vi "sample4(Multi).vi"() -> ()   [LabVIEW 2011]
uses:
  <vilib>/Platform/TimedLoop/XDataNode/timing_clust.ctl
  <vilib>/Platform/TimedLoop/XDataNode/nitl_modes.ctl
  <vilib>/Platform/TimedLoop/XDataNode/wakeup.ctl
  <vilib>/Platform/TimedLoop/XDataNode/XDataNode.xnode
  <vilib>/Platform/TimedLoop/XDataNode/XDNodeRunTimeDep.lvlib
panel:
  out "err":errorcluster caption="エラー出力" {"code" format="%04x"}
  in  "OffsetTime":u32=20
  in  "frequency":dbl=0.3
  in  "waveform":enum16{"sin", "square"}(ring)
  in  "Target ID":u8=1 max=253
  in  "Baudrate":u32=1000000
  in  "COM":refnum<visa-resource-name> caption="COMポート"
  in  "10/12bit":bool
  out "present load":i32
  in  "wave":bool
  out "CtrlTable":u8[](array[numeric]) format="%02x"
  out "Chart":T1(graph)
  out "STOP2":bool
  out "present position":u16
  in  "STOP":bool
  in  "goal position":u16(knob) scale=0.0..1023.0
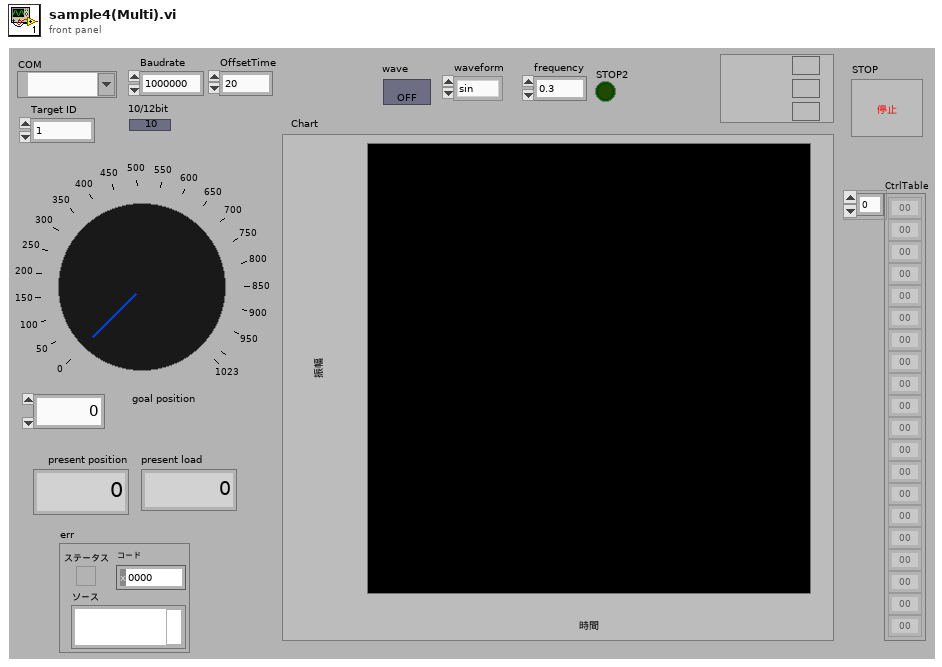
[diagram p1: front panel]
types:
  T1 = cluster{"pos":u16, "present pos":u16, "load":i32}
  T2 = typedef "XDNodeRunTimeDep.lvlib/timing_clust.ctl" = cluster{"Expected End [f-1]":u64, "Actual End [f-1]":u64, "Finished Late? [f-1]":bool, "Expected End [i-1]":u64, "Actual End [i-1]":u64, "Finished Late? [i-1]":bool, "Expected Start [i]":u64, "Actual Start [i]":u64, "Expected Start [f]":u64, "Actual Start [f]":u64, "Source Name":string, "Structure Name":string, "Period":i64, "Deadline":i64, "Offset":i64, "Start":i64, "Priority":i32, "Timeout":i32, "Mode":T3, "Wakeup Reason":T4, "Error":errorcluster, "Source Type":string, "Secondary Source Type":string, "Global End Time":u64, "Global Start Time":u64, "Frame Duration":u64, "Iteration Duration":u64, "Assigned CPU":i32, "I/O Scan Engine Mode":u32}
  T3 = typedef "XDNodeRunTimeDep.lvlib/nitl_modes.ctl" = enum32{"No Change", "Process missed periods, maintain original phase", "Discard missed periods, maintain original phase", "Process missed periods, ignore original phase", "Discard missed periods, ignore original phase"}
  T4 = typedef "XDNodeRunTimeDep.lvlib/wakeup.ctl" = enum32{"Normal", "Aborted", "Asynchronous wakeup", "Timing source error", "Timed loop error", "Timeout"}
  T5 = cluster{"goal position":u16, "present position":u16, "present load":i32}
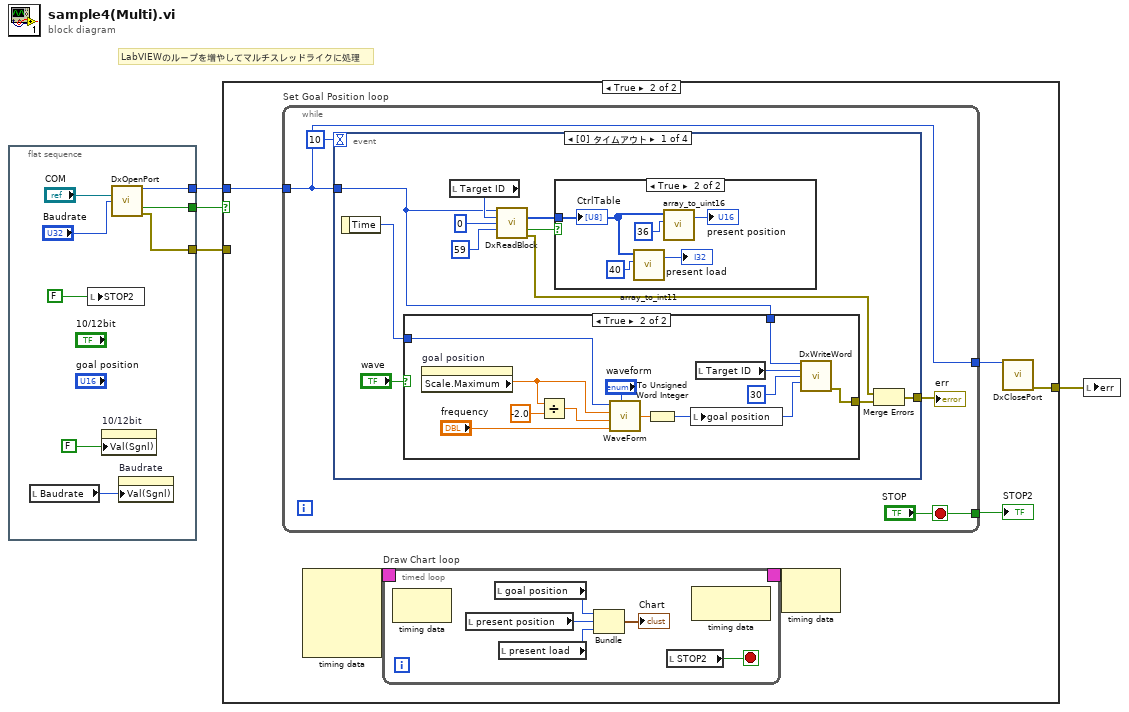
[diagram p0: block diagram]
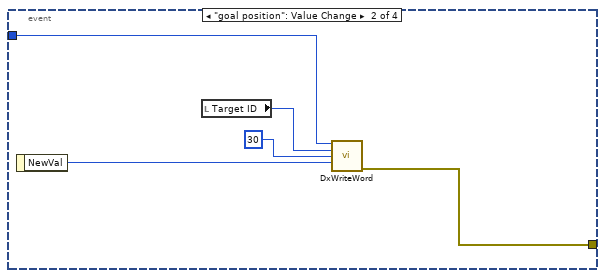
[diagram p5: hidden frame]
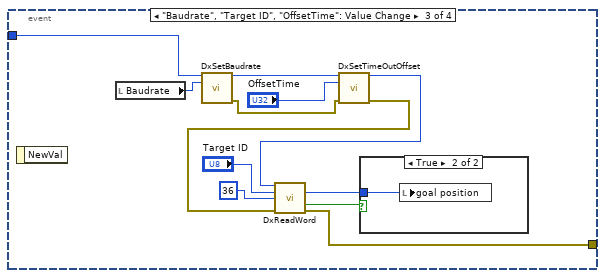
[diagram p6: hidden frame]
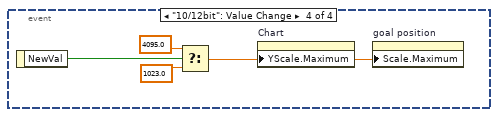
[diagram p8: hidden frame]
diagram:
  # "LabVIEWのループを増やしてマルチスレッドライクに処理"
  n1 = flat-sequence {
    tunnel: [w12] -> w4
    tunnel: [w11] -> w3
    tunnel: [w10] -> w2
    frame #0 {
      n2 = local read "Baudrate"() -> (w6:u32)
      n3 = local write "STOP2"(FALSE ("停止 3")) -> ()
      n4 = property on="10/12bit" class="Bool （指定）"("Val(Sgnl)"=FALSE ("値（信号）")) -> ()  [unwired: 2 in, 2 out]
      n5 = call "DxOpenPort.vi"("port"="COM", "baudrate"="Baudrate") -> ("dvid"=w11:u32, "成功"=w10:bool, "エラー出力"=w12:errorcluster)  [unwired: 11 in]
      n6 = property on="Baudrate" class="DigNum （指定）"("Val(Sgnl)"=w6) -> ()  [unwired: 2 in, 2 out]
    }
  }
  n7 = case shown="TRUE" w2 {
    tunnel: w4 -> [w13 _]
    tunnel: w3 -> [_ w14]
    tunnel: [w13 w15] -> w1
    frame False {
    }
    frame True {
      n8 = while "Set Goal Position loop" {
        tunnel: ["STOP"] -> w19
        tunnel: w14 -> [w31]
        tunnel: [w31] -> w18
        stop <- "STOP" stop-if-true
        n9 = event shown="[0] タイムアウト" {
          selector: _ -> [_ _ _ _]
          dyn-events: _ -> [_ _ _ _]
          timeout: 10 -> [_ _ _ _]
          tunnel: w31 -> [w36 w62 w67 _]
          tunnel: [w35 w61 w66 _] -> w30
          event Timeout {
            n10 = event-data() -> ("Time"=w38:u32)  [unwired: 1 in]
            n11 = case shown="TRUE" "wave" {
              tunnel: w38 -> [_ w46]
              tunnel: w36 -> [_ w45]
              tunnel: [_ w44] -> w34
              frame False {
              }
              frame True {
                n12 = property on="goal position" class="Knob （指定）"() -> ("Scale.Maximum"=w49:dbl)  [unwired: 2 in, 2 out]
                n13 = Divide(x=w49, y=-2.0) -> (x/y=w55:dbl)
                n14 = call "WaveForm.vi"("time(ms)"=w46, "amplitude"=w49, "offset"=w55, "frequency"="frequency", "waveform"="waveform") -> ("wave"=w51:dbl)
                n15 = To Unsigned Word Integer(number=w51) -> (unsigned 16bit integer=w50:u16)
                n16 = local write "goal position"(w50) -> ()
                n17 = local read "Target ID"() -> (w47:u8)
                n18 = call "DxWriteWord.vi"("dvid in"=w45, "id"=w47, "address"=u16 30, "data in"=w50) -> ("エラー出力"=w44:errorcluster)  [unwired: 9 in, 2 out]
              }
            }
            n19 = local read "Target ID"() -> (w43:u8)
            n20 = call "DxReadBlock.vi"("dvid in"=w36, "id"=w43, "address"=u16 0 ("pos"), "size"=u32 59) -> ("data out"=w41:u8[], "成功"=w42:bool, "エラー出力"=w33:errorcluster)  [unwired: 8 in, 1 out]
            n21 = case shown="TRUE" w42 {
              tunnel: w41 -> [_ w59]
              frame False {
              }
              frame True {
                n22 = call "array_to_int11.vi"("OffsetAddr"=u16 40 ("指標"), "array"=w59) -> ("int16"=→"present load":i16)  [unwired: 5 in]
                n23 = call "array_to_uint16.vi"("OffsetAddr"=u16 36 ("指標"), "array"=w59) -> ("uint16"=→"present position":u16)  [unwired: 5 in]
                "CtrlTable" <- w59
              }
            }
            n24 = Merge Errors(w33, w34) -> (w35:errorcluster)
          }
          event "goal position": Value Change {
            n25 = event-data() -> ("NewVal"=w63:u16)  [unwired: 1 in]
            n26 = local read "Target ID"() -> (w65:u8)
            n27 = call "DxWriteWord.vi"("dvid in"=w62, "id"=w65, "address"=u16 30, "data in"=w63) -> ("エラー出力"=w61:errorcluster)  [unwired: 9 in, 2 out]
          }
          event "Baudrate", "Target ID", "OffsetTime": Value Change {
            n28 = event-data() -> ()  [unwired: 1 in, 1 out]
            n29 = local read "Baudrate"() -> (w77:u32)
            n30 = call "DxSetBaudrate.vi"("dvid in"=w67, "Baudrate"=w77) -> ("dvid out"=w76:u32, "エラー出力"=w75:errorcluster)  [unwired: 11 in, 1 out]
            n31 = call "DxSetTimeOutOffset.vi"("dvid in"=w76, "OffsetTime"="OffsetTime", "エラー入力"=w75) -> ("dvid out"=w70:u32, "エラー出力"=w73:errorcluster)  [unwired: 11 in]
            n32 = call "DxReadWord.vi"("dvid in"=w70, "id"="Target ID", "address"=u16 36, "エラー入力"=w73) -> ("data out"=w71:u16, "成功"=w72:bool, "エラー出力"=w66:errorcluster)  [unwired: 8 in, 1 out]
            n33 = case shown="TRUE" w72 {
              tunnel: w71 -> [_ w78]
              frame False {
              }
              frame True {
                n34 = local write "goal position"(w78) -> ()
              }
            }
          }
          event "10/12bit": Value Change {
            n35 = event-data() -> ("NewVal"=w80:bool)  [unwired: 1 in]
            n36 = Select(t=4095.0 ("y"), s=w80, f=1023.0 ("y")) -> (s? t:f=w79:dbl)
            n37 = property on="Chart" class="WFChart （指定）"("YScale.Maximum"=w79) -> ()  [unwired: 2 in, 2 out]
            n38 = property on="goal position" class="Knob （指定）"("Scale.Maximum"=w79) -> ()  [unwired: 2 in, 2 out]
          }
        }
        "err" <- w30
      }
      "STOP2" <- w19
      n39 = node-c288() -> (w17:T2)  [unwired: 4 in]
      n40 = timed-loop "Draw Chart loop" {
        timing: w17 -> [_]
        timing-out: [_] -> w16
        stop <- w24 stop-if-true
        n41 = node-c288() -> ()  [unwired: 1 in, 1 out]
        n42 = local read "present position"() -> (w22:u16)
        n43 = local read "goal position"() -> (w23:u16)
        n44 = local read "present load"() -> (w20:i32)
        n45 = Bundle("goal position"=w23, "present position"=w22, "present load"=w20) -> (→"Chart":T5)  [unwired: 1 in]
        n46 = local read "STOP2"() -> (w24:bool)
        n47 = node-c288() -> ()  [unwired: 1 in, 1 out]
      }
      n48 = node-c288(w16) -> ()  [unwired: 1 out]
      n49 = call "DxClosePort.vi"("dvid"=w18) -> ("エラー出力"=w15:errorcluster)  [unwired: 13 in, 1 out]
    }
  }
  n50 = local write "err"(w1) -> ()
